vi "average from cluster.vi"() -> ()   [LabVIEW 2020]
uses:
  <vilib>/Analysis/baseanly.llb/Mean (DBL).vi
  <vilib>/Analysis/NI_AALBase.lvlib
panel:
  out "raw":dbl[][](array[numeric])
  in  "Stop":bool
  out "average":dbl[](array[numeric])
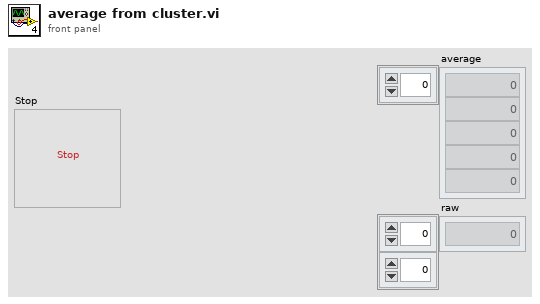
[diagram p1: front panel]
types:
  T1 = cluster{"number: 0 to 1":dbl, "number: 0 to 1":dbl, "number: 0 to 1":dbl, "number: 0 to 1":dbl, "number: 0 to 1":dbl}
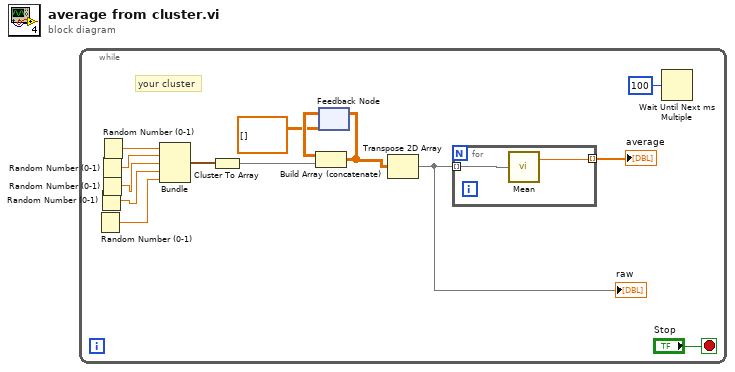
[diagram p0: block diagram]
diagram:
  n1 = while {
    stop <- "Stop" stop-if-true
    # "your cluster"
    n2 = Random Number (0-1)() -> (number: 0 to 1=w2:dbl)
    n3 = Random Number (0-1)() -> (number: 0 to 1=w3:dbl)
    n4 = Random Number (0-1)() -> (number: 0 to 1=w5:dbl)
    n5 = Random Number (0-1)() -> (number: 0 to 1=w4:dbl)
    n6 = Random Number (0-1)() -> (number: 0 to 1=w14:dbl)
    n7 = Bundle("number: 0 to 1"=w14, "number: 0 to 1"=w5, "number: 0 to 1"=w4, "number: 0 to 1"=w3, "number: 0 to 1"=w2) -> (w1:T1)  [unwired: 1 in]
    n8 = Cluster To Array(cluster=w1) -> (array=w13:dbl[])
    n9 = feedback #1(dbl[][] []) -> (w12:dbl[][])
    n10 = Build Array (concatenate)(w12, w13) -> (w8:dbl[][])
    n11 = feedback-in #1(w8) -> ()
    n12 = Transpose 2D Array(2D array=w8) -> (transposed array=w7:dbl[][])
    "raw" <- w7
    n13 = for {
      tunnel: w7 -> [w16] mode=indexing
      tunnel: [w15] -> w11 mode=indexing
      n14 = call-poly <vilib>:"Mean.vi"("X"=w16) -> ("mean"=w15:dbl)  [unwired: 1 out]
    }
    "average" <- w11
    n15 = Wait Until Next ms Multiple(millisecond multiple=u32 100) -> ()  [unwired: 1 out]
  }
